vi "TDMS interface sample.vi"() -> ()   [LabVIEW 2015]
panel:
  in  "Array 2":T1(array[cluster])
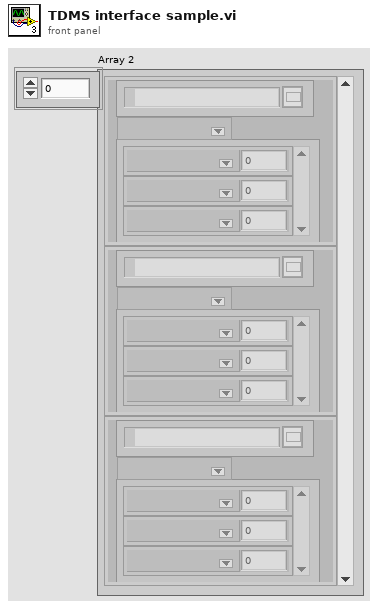
[diagram p1: front panel]
types:
  T1 = cluster{"File Path Control":path, "Array 3":cluster{"Ring":u16, "Numeric":dbl}[], "Ring":u16}[]
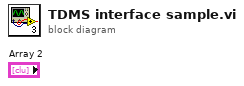
[diagram p0: block diagram]
diagram:
